vi "Clear Hardware.vi"(2 "error in (no error)":errorcluster, 3 "Arduino in":refnum<class "Arduino.lvclass">) -> (0 "error out":errorcluster, 1 "Arduino out":refnum<class "Arduino.lvclass">)   [LabVIEW 2013, in "Arduino.lvclass"]
doc: "This VI resets any necessary hardware so that the device will be ready for the next run."
uses:
  Arduino.lvclass
  Device/Device.lvclass
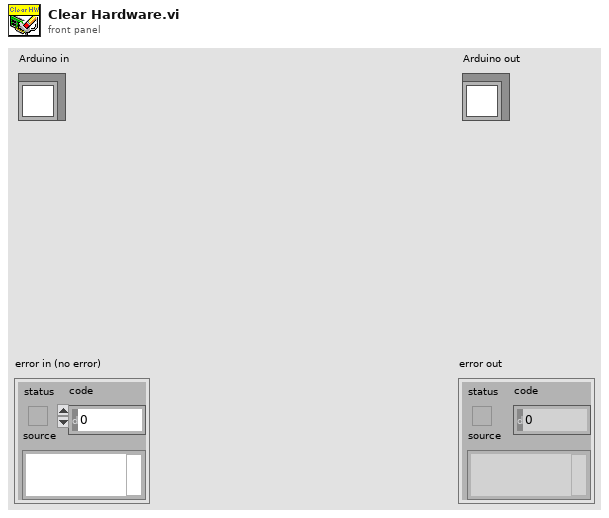
[diagram p1: front panel]
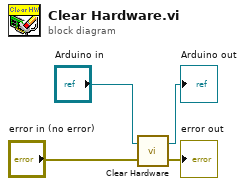
[diagram p0: block diagram]
diagram:
  n1 = call-parent "Clear Hardware.vi"("error in (no error)"="error in (no error)", "Device in"="Arduino in") -> ("error out"=→"error out":errorcluster, "Device out"=→"Arduino out":refnum<class "Arduino.lvclass">)
